vi "Read permissions.vi"(8 "error in (no error)":errorcluster, 11 "file attributes in":refnum<class "File Attributes.lvclass">) -> (0 "error out":errorcluster, 2 "permissions":u32 format="%04o", 3 "file attributes out":refnum<class "File Attributes.lvclass">)   [LabVIEW 2020, in "NI_SFTP.lvlib" / "File Attributes.lvclass"]
doc: "Returns the Unix numeric permissions information stored in this File Attributes object. These permissions are in the same form as for the <b>Get Permissions</b> function for local file I/O.\n\nThis property may not always be populated by SFTP VIs. If it does not exist, an error is returned."
uses:
  <vilib>/net/SFTP/File Attributes/File Attributes.lvclass
  <vilib>/net/SFTP/File Attributes/File Attributes.lvclass/File Attributes.ctl
  <vilib>/Utility/error.llb/Error Cluster From Error Code.vi
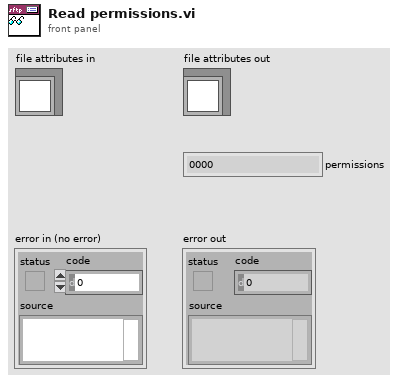
[diagram p1: front panel]
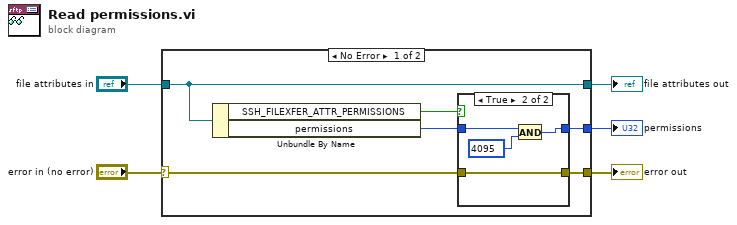
[diagram p0: block diagram]
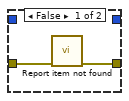
[diagram p2: hidden frame]
diagram:
  n1 = case shown="No Error" "error in (no error)" {
    selector: "error in (no error)" -> [w6 w18]
    tunnel: [w7 w18] -> w4
    tunnel: [w11 w19] -> w2
    tunnel: "file attributes in" -> [w11 w19]
    tunnel: [w9 _] -> w1
    frame No Error {
      n2 = Unbundle By Name(w11) -> ("SSH_FILEXFER_ATTR_PERMISSIONS"=w10:bool, "permissions"=w8:u32)
      n3 = case shown="True" w10 {
        tunnel: [_ w14] -> w9
        tunnel: w8 -> [_ w15]
        tunnel: [w12 w17] -> w7
        tunnel: w6 -> [w13 w17]
        frame False {
          n4 = call <vilib>:"Report item not found.vi"("error in (no error)"=w13) -> ("error out"=w12:errorcluster)  [unwired: 10 in]
        }
        frame True {
          n5 = And(x=w15, y=u32 4095) -> (x .and. y?=w14:u32)
        }
      }
    }
    frame Error {
    }
  }
  "error out" <- w4
  "file attributes out" <- w2
  "permissions" <- w1
